vi "ESTTL_Pulse_Gen_Simple.vi"(0 "Channel Enable 1":bool, 1 "Channel Enable 2":bool, 2 "Channel Enable 3":bool, 3 "Channel Enable 4":bool, 4 "Channel Enable 5":bool, 5 "Channel Enable 6":bool, 6 "Channel Enable 7":bool, 7 "Channel Enable 8":bool, 8 "ESTTL_Config":T3, 10 "FuelSparkSupervisor":T2, 14 "ESTTL.Sequence":T1, 16 "key":u16) -> (20 "CmdOut1":bool, 21 "CmdOut2":bool, 22 "CmdOut3":bool, 23 "CmdOut4":bool, 24 "CmdOut5":bool, 25 "CmdOut6":bool, 26 "CmdOut7":bool, 27 "CmdOut8":bool)   [LabVIEW 2015, in "ECS-FPGA.lvlib"]
uses:
  ECS-FPGA.lvlib
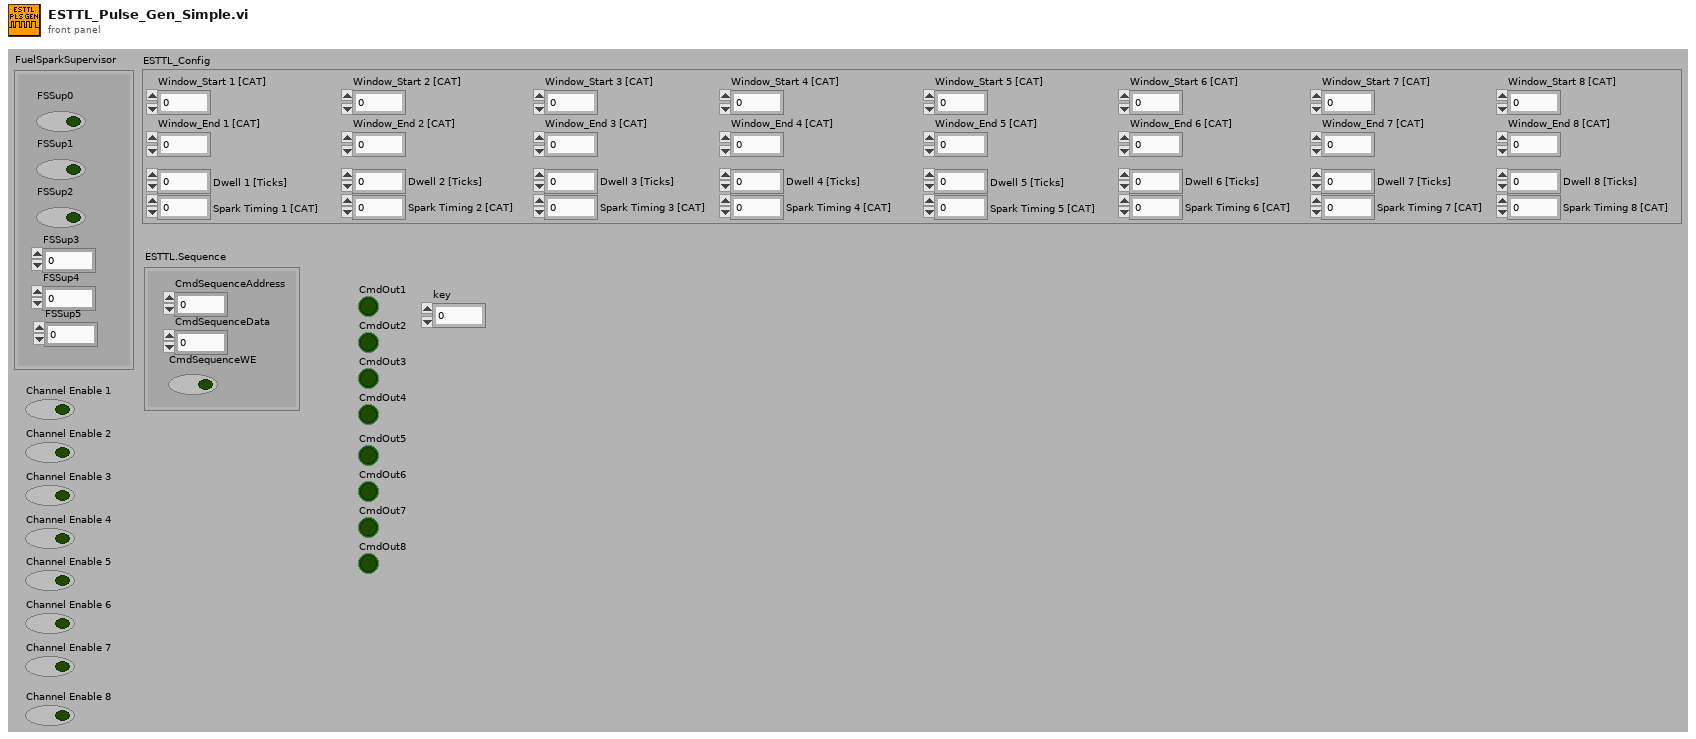
[diagram p1: front panel]
types:
  T1 = cluster{"CmdSequenceAddress":u8, "CmdSequenceData":u32, "CmdSequenceWE":bool}
  T2 = cluster{"FSSup0":bool, "FSSup1":bool, "FSSup2":bool, "FSSup3":u16, "FSSup4":u32, "FSSup5":u16}
  T3 = cluster{"Window_Start 1 [CAT]":u16, "Window_End 1 [CAT]":u16, "Window_Start 2 [CAT]":u16, "Window_End 2 [CAT]":u16, "Window_Start 3 [CAT]":u16, "Window_End 3 [CAT]":u16, "Window_Start 4 [CAT]":u16, "Window_End 4 [CAT]":u16, "Dwell 1 [Ticks]":u32, "Spark Timing 1 [CAT]":u16, "Dwell 2 [Ticks]":u32, "Spark Timing 2 [CAT]":u16, "Dwell 3 [Ticks]":u32, "Spark Timing 3 [CAT]":u16, "Dwell 4 [Ticks]":u32, "Spark Timing 4 [CAT]":u16, "Window_End 5 [CAT]":u16, "Window_Start 5 [CAT]":u16, "Window_End 6 [CAT]":u16, "Window_Start 6 [CAT]":u16, "Window_End 7 [CAT]":u16, "Window_Start 7 [CAT]":u16, "Spark Timing 5 [CAT]":u16, "Dwell 5 [Ticks]":u32, "Spark Timing 6 [CAT]":u16, "Dwell 6 [Ticks]":u32, "Spark Timing 7 [CAT]":u16, "Dwell 7 [Ticks]":u32, "Window_End 8 [CAT]":u16, "Window_Start 8 [CAT]":u16, "Spark Timing 8 [CAT]":u16, "Dwell 8 [Ticks]":u32}
  T4 = cluster{"Enable":bool, "OSAdvance":u32, "OSPosition":u16}
  T5 = cluster{"Enable":bool, "StartPosition":u16, "EndPosition":u16}
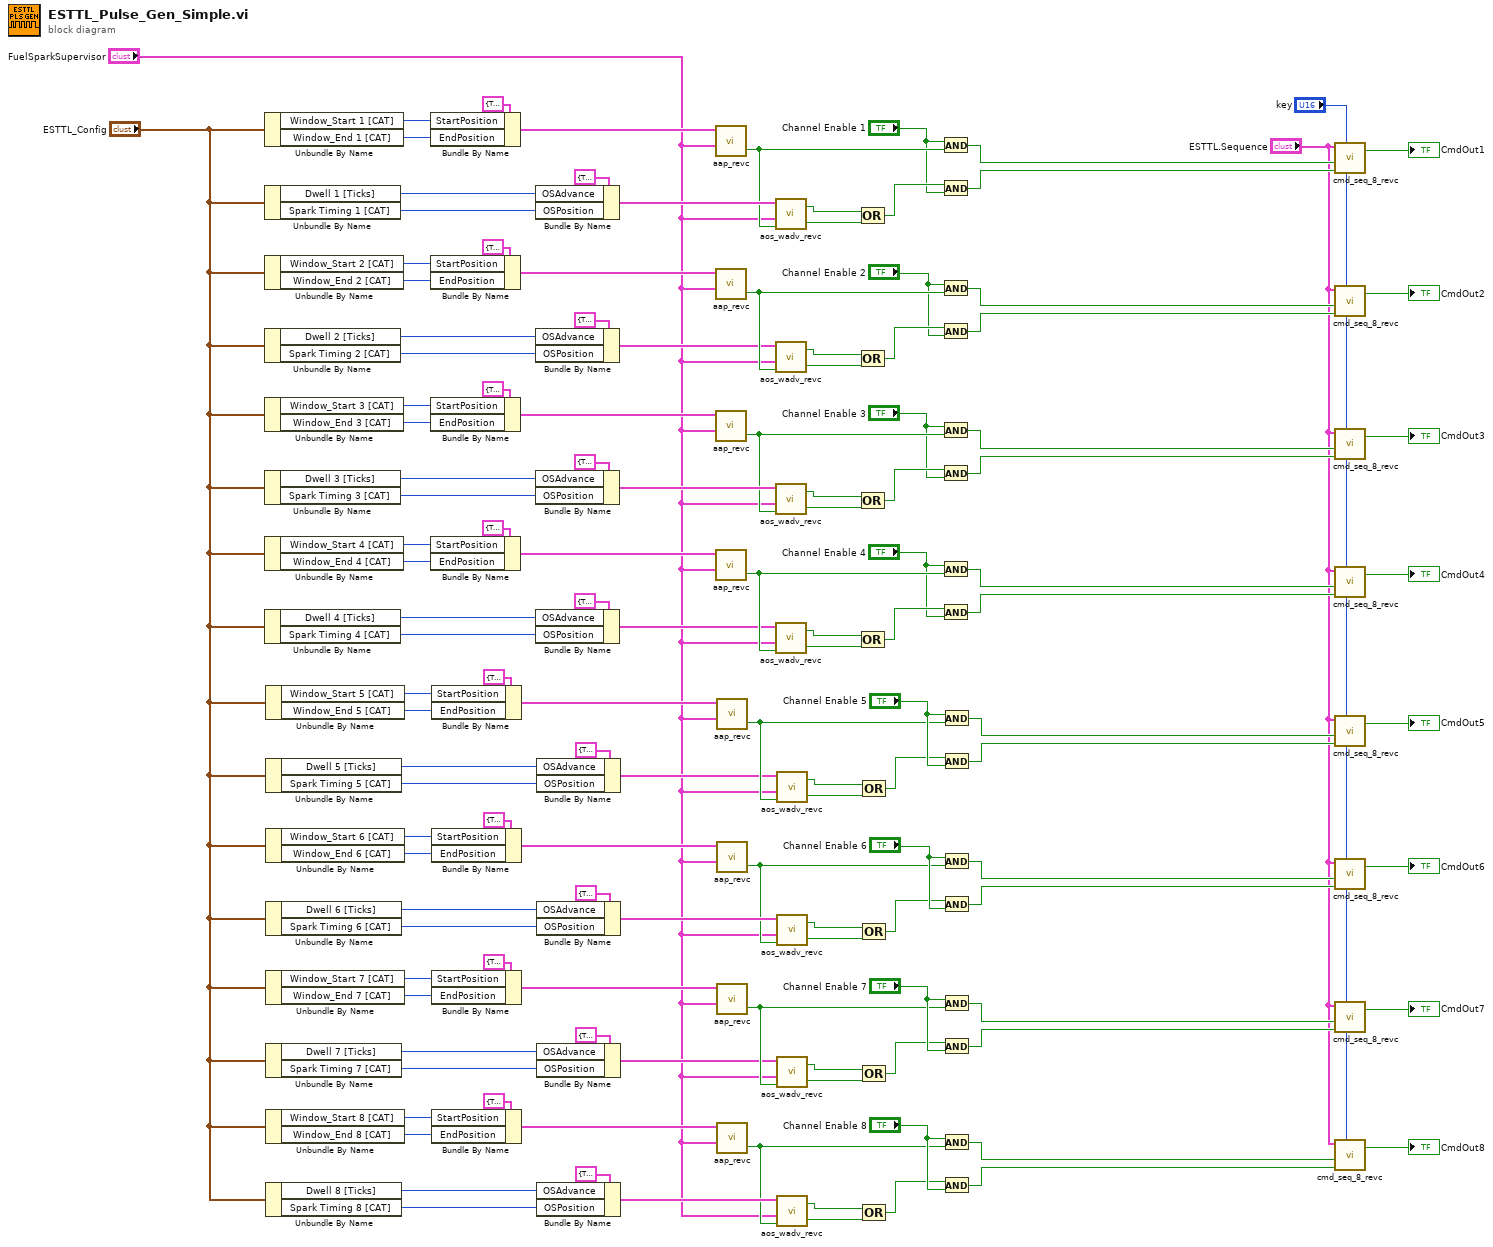
[diagram p0: block diagram]
diagram:
  n1 = Unbundle By Name("ESTTL_Config") -> ("Window_Start 1 [CAT]"=w129:u16, "Window_End 1 [CAT]"=w128:u16)
  n2 = Unbundle By Name("ESTTL_Config") -> ("Dwell 1 [Ticks]"=w126:u32, "Spark Timing 1 [CAT]"=w122:u16)
  n3 = Unbundle By Name("ESTTL_Config") -> ("Window_Start 2 [CAT]"=w115:u16, "Window_End 2 [CAT]"=w116:u16)
  n4 = Unbundle By Name("ESTTL_Config") -> ("Dwell 2 [Ticks]"=w118:u32, "Spark Timing 2 [CAT]"=w121:u16)
  n5 = Unbundle By Name("ESTTL_Config") -> ("Window_Start 3 [CAT]"=w107:u16, "Window_End 3 [CAT]"=w106:u16)
  n6 = Unbundle By Name("ESTTL_Config") -> ("Dwell 3 [Ticks]"=w104:u32, "Spark Timing 3 [CAT]"=w101:u16)
  n7 = Unbundle By Name("ESTTL_Config") -> ("Window_Start 4 [CAT]"=w93:u16, "Window_End 4 [CAT]"=w94:u16)
  n8 = Unbundle By Name("ESTTL_Config") -> ("Dwell 4 [Ticks]"=w96:u32, "Spark Timing 4 [CAT]"=w99:u16)
  n9 = Unbundle By Name("ESTTL_Config") -> ("Window_Start 5 [CAT]"=w8:u16, "Window_End 5 [CAT]"=w9:u16)
  n10 = Unbundle By Name("ESTTL_Config") -> ("Dwell 5 [Ticks]"=w11:u32, "Spark Timing 5 [CAT]"=w15:u16)
  n11 = Unbundle By Name("ESTTL_Config") -> ("Window_Start 6 [CAT]"=w22:u16, "Window_End 6 [CAT]"=w21:u16)
  n12 = Unbundle By Name("ESTTL_Config") -> ("Dwell 6 [Ticks]"=w19:u32, "Spark Timing 6 [CAT]"=w16:u16)
  n13 = Unbundle By Name("ESTTL_Config") -> ("Window_Start 7 [CAT]"=w30:u16, "Window_End 7 [CAT]"=w31:u16)
  n14 = Unbundle By Name("ESTTL_Config") -> ("Dwell 7 [Ticks]"=w33:u32, "Spark Timing 7 [CAT]"=w36:u16)
  n15 = Unbundle By Name("ESTTL_Config") -> ("Window_Start 8 [CAT]"=w44:u16, "Window_End 8 [CAT]"=w43:u16)
  n16 = Unbundle By Name("ESTTL_Config") -> ("Dwell 8 [Ticks]"=w41:u32, "Spark Timing 8 [CAT]"=w38:u16)
  n17 = Bundle By Name(cluster=T5 {"Enable"=TRUE, "StartPosition"=0, "EndPosition"=0} ("OP Windiw Definition"), "StartPosition"=w129, "EndPosition"=w128) -> (w131:T5)
  n18 = Bundle By Name(cluster=T5 {"Enable"=TRUE, "StartPosition"=0, "EndPosition"=0} ("OP Windiw Definition"), "StartPosition"=w115, "EndPosition"=w116) -> (w113:T5)
  n19 = Bundle By Name(cluster=T5 {"Enable"=TRUE, "StartPosition"=0, "EndPosition"=0} ("OP Windiw Definition"), "StartPosition"=w107, "EndPosition"=w106) -> (w109:T5)
  n20 = Bundle By Name(cluster=T5 {"Enable"=TRUE, "StartPosition"=0, "EndPosition"=0} ("OP Windiw Definition"), "StartPosition"=w93, "EndPosition"=w94) -> (w91:T5)
  n21 = Bundle By Name(cluster=T5 {"Enable"=TRUE, "StartPosition"=0, "EndPosition"=0} ("OP Windiw Definition"), "StartPosition"=w8, "EndPosition"=w9) -> (w6:T5)
  n22 = Bundle By Name(cluster=T5 {"Enable"=TRUE, "StartPosition"=0, "EndPosition"=0} ("OP Windiw Definition"), "StartPosition"=w22, "EndPosition"=w21) -> (w24:T5)
  n23 = Bundle By Name(cluster=T5 {"Enable"=TRUE, "StartPosition"=0, "EndPosition"=0} ("OP Windiw Definition"), "StartPosition"=w30, "EndPosition"=w31) -> (w28:T5)
  n24 = Bundle By Name(cluster=T5 {"Enable"=TRUE, "StartPosition"=0, "EndPosition"=0} ("OP Windiw Definition"), "StartPosition"=w44, "EndPosition"=w43) -> (w46:T5)
  n25 = Bundle By Name(cluster=T4 {"Enable"=TRUE, "OSAdvance"=0, "OSPosition"=0} ("AOSControl"), "OSAdvance"=w126, "OSPosition"=w122) -> (w132:T4)
  n26 = Bundle By Name(cluster=T4 {"Enable"=TRUE, "OSAdvance"=0, "OSPosition"=0} ("AOSControl"), "OSAdvance"=w118, "OSPosition"=w121) -> (w112:T4)
  n27 = Bundle By Name(cluster=T4 {"Enable"=TRUE, "OSAdvance"=0, "OSPosition"=0} ("AOSControl"), "OSAdvance"=w104, "OSPosition"=w101) -> (w110:T4)
  n28 = Bundle By Name(cluster=T4 {"Enable"=TRUE, "OSAdvance"=0, "OSPosition"=0} ("AOSControl"), "OSAdvance"=w96, "OSPosition"=w99) -> (w90:T4)
  n29 = Bundle By Name(cluster=T4 {"Enable"=TRUE, "OSAdvance"=0, "OSPosition"=0} ("AOSControl"), "OSAdvance"=w11, "OSPosition"=w15) -> (w5:T4)
  n30 = Bundle By Name(cluster=T4 {"Enable"=TRUE, "OSAdvance"=0, "OSPosition"=0} ("AOSControl"), "OSAdvance"=w19, "OSPosition"=w16) -> (w25:T4)
  n31 = Bundle By Name(cluster=T4 {"Enable"=TRUE, "OSAdvance"=0, "OSPosition"=0} ("AOSControl"), "OSAdvance"=w33, "OSPosition"=w36) -> (w27:T4)
  n32 = Bundle By Name(cluster=T4 {"Enable"=TRUE, "OSAdvance"=0, "OSPosition"=0} ("AOSControl"), "OSAdvance"=w41, "OSPosition"=w38) -> (w47:T4)
  n33 = call <vilib>:"aap_revc.vi"("FuelSparkSupervisor"="FuelSparkSupervisor", "AAPControl"=w131) -> ("AAP"=w125:bool)  [unwired: 3 in]
  n34 = call <vilib>:"aap_revc.vi"("FuelSparkSupervisor"="FuelSparkSupervisor", "AAPControl"=w113) -> ("AAP"=w119:bool)  [unwired: 3 in]
  n35 = call <vilib>:"aap_revc.vi"("FuelSparkSupervisor"="FuelSparkSupervisor", "AAPControl"=w109) -> ("AAP"=w103:bool)  [unwired: 3 in]
  n36 = call <vilib>:"aap_revc.vi"("FuelSparkSupervisor"="FuelSparkSupervisor", "AAPControl"=w91) -> ("AAP"=w97:bool)  [unwired: 3 in]
  n37 = call <vilib>:"aap_revc.vi"("FuelSparkSupervisor"="FuelSparkSupervisor", "AAPControl"=w6) -> ("AAP"=w12:bool)  [unwired: 3 in]
  n38 = call <vilib>:"aap_revc.vi"("FuelSparkSupervisor"="FuelSparkSupervisor", "AAPControl"=w24) -> ("AAP"=w18:bool)  [unwired: 3 in]
  n39 = call <vilib>:"aap_revc.vi"("FuelSparkSupervisor"="FuelSparkSupervisor", "AAPControl"=w28) -> ("AAP"=w34:bool)  [unwired: 3 in]
  n40 = call <vilib>:"aap_revc.vi"("FuelSparkSupervisor"="FuelSparkSupervisor", "AAPControl"=w46) -> ("AAP"=w40:bool)  [unwired: 3 in]
  n41 = call <vilib>:"aos_wadv_revc.vi"("OpWindow"=w125, "FuelSparkSupervisor"="FuelSparkSupervisor", "AOSControl"=w132) -> ("AOS"=w72:bool, "AOSAdv"=w76:bool)  [unwired: 1 in]
  n42 = call <vilib>:"aos_wadv_revc.vi"("OpWindow"=w119, "FuelSparkSupervisor"="FuelSparkSupervisor", "AOSControl"=w112) -> ("AOS"=w71:bool, "AOSAdv"=w75:bool)  [unwired: 1 in]
  n43 = call <vilib>:"aos_wadv_revc.vi"("OpWindow"=w103, "FuelSparkSupervisor"="FuelSparkSupervisor", "AOSControl"=w110) -> ("AOS"=w70:bool, "AOSAdv"=w74:bool)  [unwired: 1 in]
  n44 = call <vilib>:"aos_wadv_revc.vi"("OpWindow"=w97, "FuelSparkSupervisor"="FuelSparkSupervisor", "AOSControl"=w90) -> ("AOS"=w69:bool, "AOSAdv"=w73:bool)  [unwired: 1 in]
  n45 = call <vilib>:"aos_wadv_revc.vi"("OpWindow"=w12, "FuelSparkSupervisor"="FuelSparkSupervisor", "AOSControl"=w5) -> ("AOS"=w65:bool, "AOSAdv"=w61:bool)  [unwired: 1 in]
  n46 = call <vilib>:"aos_wadv_revc.vi"("OpWindow"=w18, "FuelSparkSupervisor"="FuelSparkSupervisor", "AOSControl"=w25) -> ("AOS"=w66:bool, "AOSAdv"=w62:bool)  [unwired: 1 in]
  n47 = call <vilib>:"aos_wadv_revc.vi"("OpWindow"=w34, "FuelSparkSupervisor"="FuelSparkSupervisor", "AOSControl"=w27) -> ("AOS"=w67:bool, "AOSAdv"=w63:bool)  [unwired: 1 in]
  n48 = call <vilib>:"aos_wadv_revc.vi"("OpWindow"=w40, "FuelSparkSupervisor"="FuelSparkSupervisor", "AOSControl"=w47) -> ("AOS"=w68:bool, "AOSAdv"=w64:bool)  [unwired: 1 in]
  n49 = Compound Arithmetic op=OR(w76, w72) -> (w127:bool)
  n50 = Compound Arithmetic op=OR(w75, w71) -> (w117:bool)
  n51 = Compound Arithmetic op=OR(w74, w70) -> (w105:bool)
  n52 = Compound Arithmetic op=OR(w73, w69) -> (w95:bool)
  n53 = Compound Arithmetic op=OR(w61, w65) -> (w10:bool)
  n54 = Compound Arithmetic op=OR(w62, w66) -> (w20:bool)
  n55 = Compound Arithmetic op=OR(w63, w67) -> (w32:bool)
  n56 = Compound Arithmetic op=OR(w64, w68) -> (w42:bool)
  n57 = And(x="Channel Enable 1", y=w125) -> (x .and. y?=w87:bool)
  n58 = And(x=w127, y="Channel Enable 1") -> (x .and. y?=w88:bool)
  n59 = And(x="Channel Enable 2", y=w119) -> (x .and. y?=w85:bool)
  n60 = And(x=w117, y="Channel Enable 2") -> (x .and. y?=w84:bool)
  n61 = And(x="Channel Enable 3", y=w103) -> (x .and. y?=w82:bool)
  n62 = And(x=w105, y="Channel Enable 3") -> (x .and. y?=w81:bool)
  n63 = And(x="Channel Enable 4", y=w97) -> (x .and. y?=w79:bool)
  n64 = And(x=w95, y="Channel Enable 4") -> (x .and. y?=w78:bool)
  n65 = And(x="Channel Enable 5", y=w12) -> (x .and. y?=w50:bool)
  n66 = And(x=w10, y="Channel Enable 5") -> (x .and. y?=w49:bool)
  n67 = And(x="Channel Enable 6", y=w18) -> (x .and. y?=w52:bool)
  n68 = And(x=w20, y="Channel Enable 6") -> (x .and. y?=w53:bool)
  n69 = And(x="Channel Enable 7", y=w34) -> (x .and. y?=w55:bool)
  n70 = And(x=w32, y="Channel Enable 7") -> (x .and. y?=w56:bool)
  n71 = And(x="Channel Enable 8", y=w40) -> (x .and. y?=w58:bool)
  n72 = And(x=w42, y="Channel Enable 8") -> (x .and. y?=w59:bool)
  n73 = call <vilib>:"cmd_seq_8_revc.vi"("CmdSequencePort"="ESTTL.Sequence", "SequenceReset"=w87, "Trigger"=w88, "key"="key") -> ("Command"=→"CmdOut1":bool)  [unwired: 1 in, 1 out]
  n74 = call <vilib>:"cmd_seq_8_revc.vi"("CmdSequencePort"="ESTTL.Sequence", "SequenceReset"=w85, "Trigger"=w84, "key"="key") -> ("Command"=→"CmdOut2":bool)  [unwired: 1 in, 1 out]
  n75 = call <vilib>:"cmd_seq_8_revc.vi"("CmdSequencePort"="ESTTL.Sequence", "SequenceReset"=w82, "Trigger"=w81, "key"="key") -> ("Command"=→"CmdOut3":bool)  [unwired: 1 in, 1 out]
  n76 = call <vilib>:"cmd_seq_8_revc.vi"("CmdSequencePort"="ESTTL.Sequence", "SequenceReset"=w79, "Trigger"=w78, "key"="key") -> ("Command"=→"CmdOut4":bool)  [unwired: 1 in, 1 out]
  n77 = call <vilib>:"cmd_seq_8_revc.vi"("CmdSequencePort"="ESTTL.Sequence", "SequenceReset"=w50, "Trigger"=w49, "key"="key") -> ("Command"=→"CmdOut5":bool)  [unwired: 1 in, 1 out]
  n78 = call <vilib>:"cmd_seq_8_revc.vi"("CmdSequencePort"="ESTTL.Sequence", "SequenceReset"=w52, "Trigger"=w53, "key"="key") -> ("Command"=→"CmdOut6":bool)  [unwired: 1 in, 1 out]
  n79 = call <vilib>:"cmd_seq_8_revc.vi"("CmdSequencePort"="ESTTL.Sequence", "SequenceReset"=w55, "Trigger"=w56, "key"="key") -> ("Command"=→"CmdOut7":bool)  [unwired: 1 in, 1 out]
  n80 = call <vilib>:"cmd_seq_8_revc.vi"("CmdSequencePort"="ESTTL.Sequence", "SequenceReset"=w58, "Trigger"=w59, "key"="key") -> ("Command"=→"CmdOut8":bool)  [unwired: 1 in, 1 out]
